vi "String.vi"() -> ()   [LabVIEW 2020]
panel:
  out "concatenated string 3":string
  in  "Boolean 2":bool
  in  "Tank":u32(slide) scale=0.0..10.0
  in  "Thermometer":dbl(slide) scale=0.0..100.0
  in  "Boolean":bool
  out "concatenated string 2":string
  in  "Indique su nombre":string
  in  "Indique Apellido":string
  out "all lower case string":string
  out "all upper case string":string
  out "substring":string
  in  "length (rest)":i32
  in  "offset (0)":i32
  out "concatenated string":string
  out "length":i32
  out "Dato B":string
  in  "Dato A":string
  # "String"
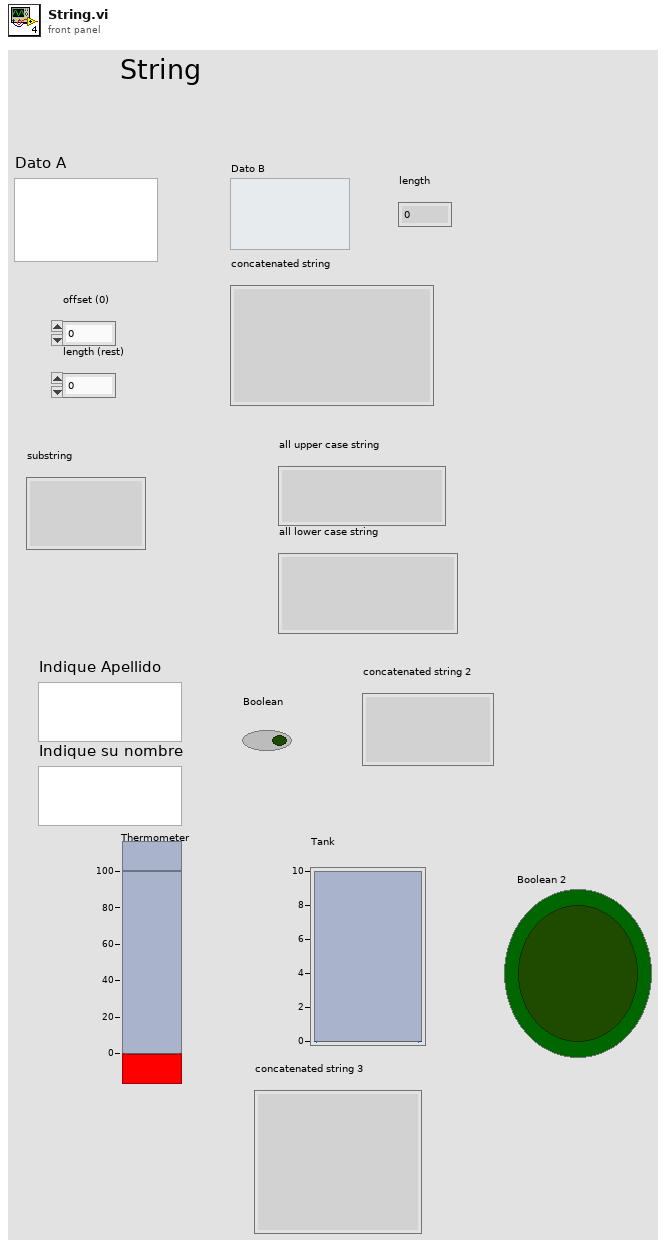
[diagram p1: front panel]
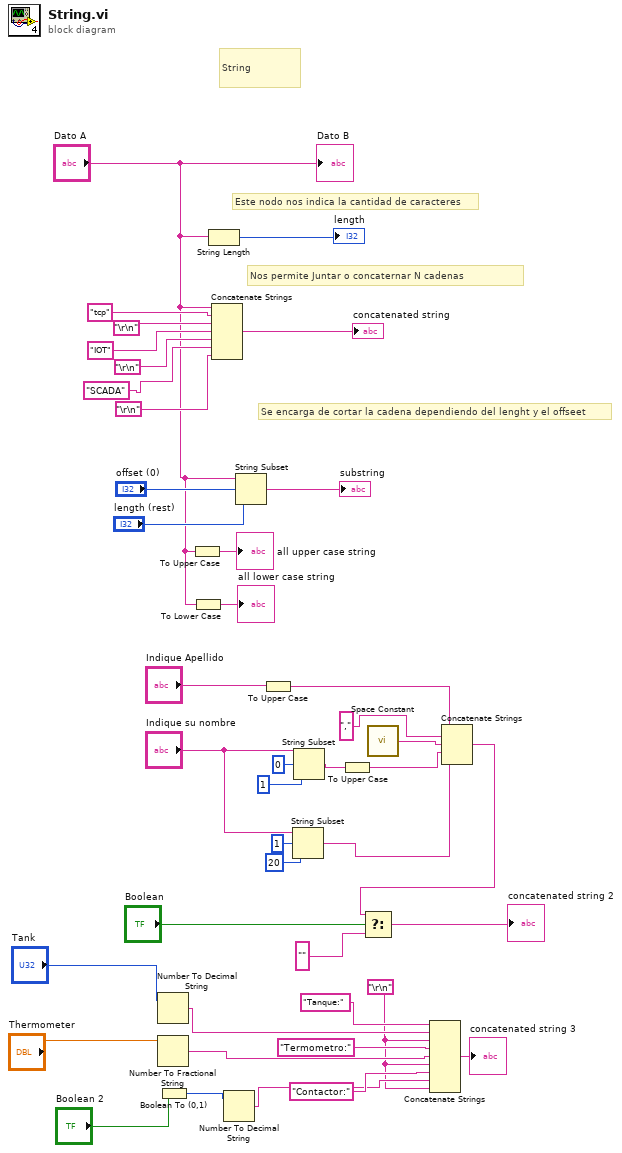
[diagram p0: block diagram]
diagram:
  w2 = "\r\n"
  # "Se encarga de cortar la cadena dependiendo del lenght y el offseet"
  # "Nos permite Juntar o concaternar N cadenas"
  # "Este nodo nos indica la cantidad de caracteres"
  # "String"
  n1 = Number To Decimal String(number="Tank") -> (decimal integer string=w7:string)  [unwired: 1 in]
  n2 = Number To Fractional String(number="Thermometer") -> (F-format string=w5:string)  [unwired: 3 in]
  n3 = Boolean To (0,1)(Boolean="Boolean 2") -> (0, 1=w9:i16)
  n4 = To Upper Case(1:"Dato A") -> (0:→"all upper case string":string)
  n5 = To Lower Case(string="Dato A") -> (all lower case string=→"all lower case string":string)
  n6 = String Length(string="Dato A") -> (length=→"length":i32)
  n7 = Concatenate Strings("Dato A", "tcp", "\r\n", "IOT", "\r\n", "SCADA", "\r\n") -> (→"concatenated string":string)
  n8 = Number To Decimal String(number=w9) -> (decimal integer string=w3:string)  [unwired: 1 in]
  n9 = String Subset(string="Dato A", offset (0)="offset (0)", length (rest)="length (rest)") -> (substring=→"substring":string)
  n10 = To Upper Case(1:"Indique Apellido") -> (0:w22:string)
  n11 = String Subset(string="Indique su nombre", offset (0)=1, length (rest)=20 ("length (rest)")) -> (substring=w19:string)
  n12 = String Subset(string="Indique su nombre", offset (0)=0, length (rest)=1 ("length (rest)")) -> (substring=w18:string)
  n13 = To Upper Case(1:w18) -> (0:w17:string)
  n14 = call <vilib>:"Space Constant.vi"() -> ("String"=w20:string)
  n15 = Concatenate Strings("Tanque:", w7, w2, "Termometro:", w5, w2, "Contactor:", w3, w2) -> (→"concatenated string 3":string)
  n16 = Concatenate Strings(w22, ",", w20, w17, w19) -> (w14:string)
  n17 = Select(t=w14, s="Boolean", f="") -> (s? t:f=→"concatenated string 2":string)
  "Dato B" <- "Dato A"
